vi "get_image.vi"(7 "get image as...":T1, 8 "error in (no error)":errorcluster, 10 "index":i32, 11 "ImageCollection in":refnum<class "ImageCollection.lvclass">) -> (0 "error out":errorcluster, 2 "Image.lvclass":refnum<class "Image.lvclass">, 3 "ImageCollection out":refnum<class "ImageCollection.lvclass">)   [LabVIEW 2010, in "ImageCollection.lvclass"]
uses:
  ImageCollection.lvclass
  Image/Image/Image.lvclass
  add_mode_enum.ctl
  ImageCollection.lvclass/ImageCollection.ctl
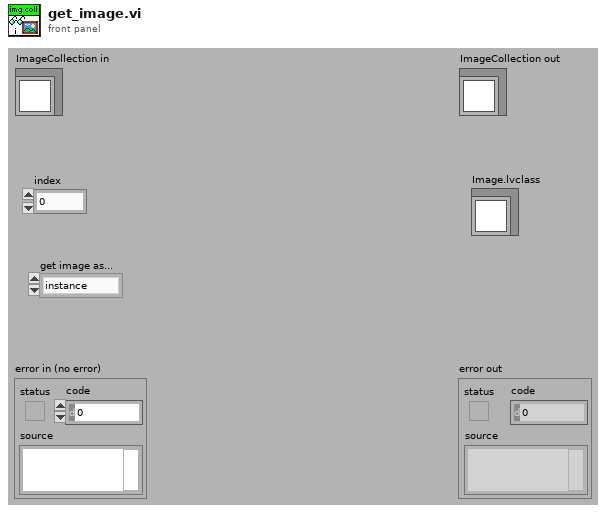
[diagram p1: front panel]
types:
  T1 = typedef "ImageCollection.lvclass/add_mode_enum.ctl" = enum16{"instance", "copy"}
  T2 = typedef "ImageCollection.lvclass/storage_mode_enum.ctl" = enum16{"RAM", "single files", "multipage TIFF (read-only)"}
  T3 = typedef "Image Type" = u32
  T4 = typedef "Image.lvclass/storage_mode.ctl" = enum16{"RAM", "disk"}
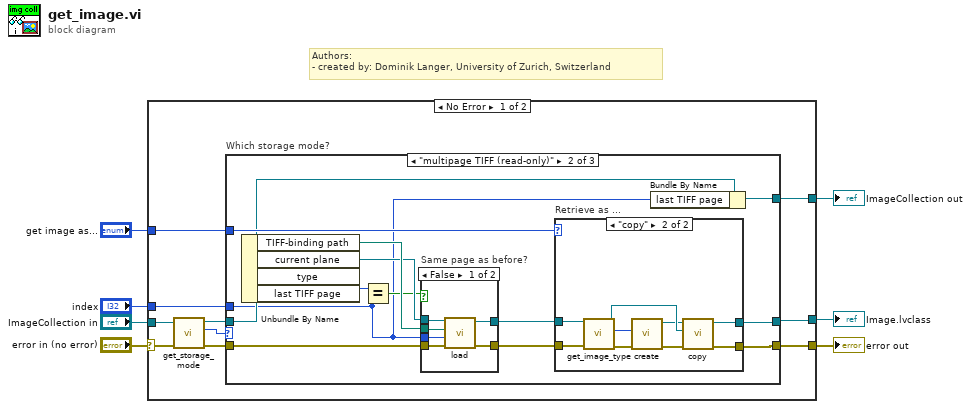
[diagram p0: block diagram]
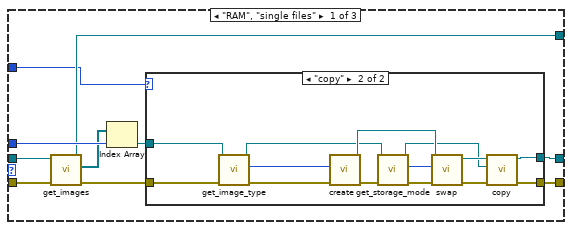
[diagram p2: hidden frame]
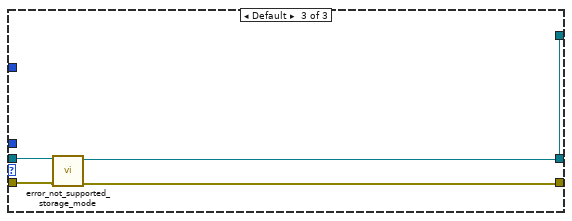
[diagram p6: hidden frame]
diagram:
  # "Authors: \n- created by: Dominik Langer, University of Zurich, Switzerland"
  n1 = case shown="No Error" "error in (no error)" {
    selector: "error in (no error)" -> [w17 w81]
    tunnel: [w12 w81] -> w6
    tunnel: [w8 w80] -> w4
    tunnel: "ImageCollection in" -> [w16 w80]
    tunnel: [w11 _] -> w3
    tunnel: "index" -> [w9 _]
    tunnel: "get image as..." -> [w13 _]
    frame No Error {
      n2 = call-dynamic "get_storage_mode.vi"("error in (no error)"=w17, "ImageCollection.lvclass in"=w16) -> ("error out"=w14:errorcluster, "storage type"=w15:T2, "ImageCollection.lvclass out"=w10:refnum<class "ImageCollection.lvclass">)  [unwired: 7 out]
      n3 = case "Which storage mode?" shown="\"multipage TIFF (read-only)\"" w15 {
        tunnel: w14 -> [w25 w55 w79]
        tunnel: w9 -> [w27 w44 _]
        tunnel: [w21 w51 _] -> w11
        tunnel: [w22 w52 w78] -> w12
        tunnel: w10 -> [w26 w46 w77]
        tunnel: [w23 w45 w76] -> w8
        tunnel: w13 -> [w18 w50 _]
        frame "RAM", "single files" {
          n4 = call-dynamic "get_images.vi"("error in (no error)"=w25, "ImageCollection.lvclass in"=w26) -> ("error out"=w19:errorcluster, "images"=w24:refnum<class "Image.lvclass">[], "ImageCollection.lvclass out"=w23:refnum<class "ImageCollection.lvclass">)  [unwired: 7 out]
          n5 = Index Array(array=w24, index=w27) -> (element=w20:refnum<class "Image.lvclass">)
          n6 = case shown="\"copy\"" w18 {
            tunnel: [w28 w43] -> w22
            tunnel: [w29 w42] -> w21
            tunnel: w20 -> [w29 w32]
            tunnel: w19 -> [w28 w30]
            frame "instance", Default {
            }
            frame "copy" {
              n7 = call-dynamic "get_image_type.vi"("error in (no error)"=w30, "Image.lvclass in"=w32) -> ("error out"=w40:errorcluster, "Image Type"=w41:T3, "Image.lvclass out"=w31:refnum<class "Image.lvclass">)  [unwired: 7 out]
              n8 = call "create.vi"("error in (no error)"=w40, "Image Type"=w41) -> ("error out"=w36:errorcluster, "Image out"=w39:refnum<class "Image.lvclass">)  [unwired: 2 in, 6 out]
              n9 = call-dynamic "get_storage_mode.vi"("error in (no error)"=w36, "Image.lvclass in"=w31) -> ("error out"=w34:errorcluster, "storage mode"=w33:T4, "Image.lvclass out"=w35:refnum<class "Image.lvclass">)  [unwired: 7 out]
              n10 = call-dynamic "swap.vi"("error in (no error)"=w34, "storage type target"=w33, "Image in"=w39) -> ("error out"=w38:errorcluster, "Image out"=w37:refnum<class "Image.lvclass">)  [unwired: 7 out]
              n11 = call "copy.vi"("error in (no error)"=w38, "image to copy (source)"=w35, "Image in (target)"=w37) -> ("error out"=w43:errorcluster, "Image out"=w42:refnum<class "Image.lvclass">)  [unwired: 7 out]
            }
          }
        }
        frame "multipage TIFF (read-only)" {
          n12 = Unbundle By Name(w46) -> ("TIFF-binding path"=w56:path, "current plane"=w54:refnum<class "Image.lvclass">, "last TIFF page"=w48:i32)  [unwired: 1 out]
          n13 = Equal?(x=w48, y=w44) -> (x = y?=w47:bool)
          n14 = case "Same page as before?" shown="False" w47 {
            tunnel: w56 -> [w62 _]
            tunnel: w55 -> [w61 w64]
            tunnel: w54 -> [w60 w63]
            tunnel: [w59 w64] -> w53
            tunnel: [w58 w63] -> w49
            tunnel: w44 -> [w57 _]
            frame False {
              n15 = call-dynamic "load.vi"("error in (no error)"=w61, "page"=w57, "Path"=w62, "Image in"=w60) -> ("error out"=w59:errorcluster, "Image out"=w58:refnum<class "Image.lvclass">)  [unwired: 4 in, 2 out]
            }
            frame True {
            }
          }
          n16 = case "Retrieve as ..." shown="\"copy\"" w50 {
            tunnel: w53 -> [w66 w75]
            tunnel: [w66 w71] -> w52
            tunnel: [w65 w70] -> w51
            tunnel: w49 -> [w65 w69]
            frame "instance", Default {
            }
            frame "copy" {
              n17 = call-dynamic "get_image_type.vi"("error in (no error)"=w75, "Image.lvclass in"=w69) -> ("error out"=w74:errorcluster, "Image Type"=w73:T3, "Image.lvclass out"=w68:refnum<class "Image.lvclass">)  [unwired: 7 out]
              n18 = call "create.vi"("error in (no error)"=w74, "Image Type"=w73) -> ("error out"=w72:errorcluster, "Image out"=w67:refnum<class "Image.lvclass">)  [unwired: 2 in, 6 out]
              n19 = call "copy.vi"("error in (no error)"=w72, "image to copy (source)"=w68, "Image in (target)"=w67) -> ("error out"=w71:errorcluster, "Image out"=w70:refnum<class "Image.lvclass">)  [unwired: 7 out]
            }
          }
          n20 = Bundle By Name(cluster=w46, "last TIFF page"=w44) -> (w45:refnum<class "ImageCollection.lvclass">)
        }
        frame Default {
          n21 = call-dynamic "error_not_supported_storage_mode.vi"("error in (no error)"=w79, "ImageCollection in"=w77) -> ("error out"=w78:errorcluster, "ImageCollection out"=w76:refnum<class "ImageCollection.lvclass">)  [unwired: 8 out]
        }
      }
    }
    frame Error {
    }
  }
  "error out" <- w6
  "ImageCollection out" <- w4
  "Image.lvclass" <- w3
